vi "Next JSON Value.vi"(10 "Offset":i32, 11 "JSON":string) -> (1 "<JSON>Value":string, 2 "Offset past Value":i32, 3 "Rest of input":string, 4 "JSON Value Type":T1)   [LabVIEW 2015, in "JSONtext.lvlib"]
doc: "Gets the next JSON Value (object, array, string, number, true, false, or null)\n\n\"Offset\" should point to the start of the JSON Value, or to whitespace in front of the Value."
uses:
  JSONtext.lvlib
  JSON Value Type.ctl
  Parsing State.ctl
  Advance past whitespace.vi
  Advance past String.vi
  Advance past Number.vi
  Advance past Object.vi
  Advance past Array.vi
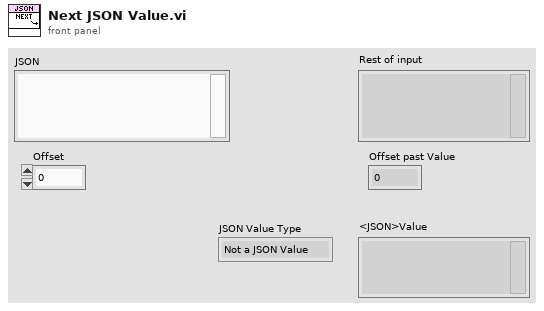
[diagram p1: front panel]
types:
  T1 = typedef "JSON Value Type.ctl" = enum16{"Not a JSON Value", "JSON Object", "JSON Array", "String", "Number", "true", "false", "null"}
  T2 = typedef "JSONtext.lvlib/Parsing State.ctl" = enum16{"Parser Error", "Object", "Array", "String", "Number/Other", "Leading Whitespace", "Object end", "Array end", "Value end"}
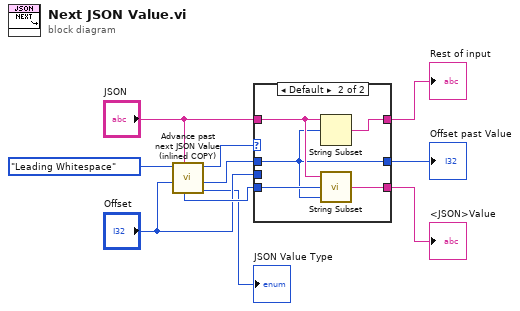
[diagram p0: block diagram]
diagram:
  n1 = call "Advance past next JSON Value (inlined COPY).vi"("JSON"="JSON", "Offset"="Offset", "State"=Parsing_State."Leading Whitespace" ("Parser State in")) -> ("JSON Value Type"=→"JSON Value Type":T1, "Offset"=w7:i32, "State"=w2:T2, "Value start"=w9:i32)  [unwired: 4 in, 1 out]
  n2 = case shown="Default" w2 {
    tunnel: w9 -> [_ w17]
    tunnel: "Offset" -> [w11 _]
    tunnel: w7 -> [_ w13]
    tunnel: [_ w16] -> w6
    tunnel: "JSON" -> [w12 w15]
    tunnel: [w12 w14] -> w3
    tunnel: [w11 w13] -> w1
    frame "Parser Error" {
    }
    frame Default {
      n3 = String Subset(string=w15, offset (0)=w13) -> (substring=w14:string)  [unwired: 1 in]
      n4 = call "String Subset.vi"("Offset past End"=w13, "Start offset"=w17, "JSON"=w15) -> ("substring"=w16:string)  [unwired: 2 in]
    }
  }
  "Rest of input" <- w3
  "<JSON>Value" <- w6
  "Offset past Value" <- w1
